vi "InsertAndPadVariantArrayBy1DIndex.vi"(9 "Array In":variant, 10 "Array Index (or -1)":i32, 11 "Value":variant) -> (3 "Reshaped VArray":variant)   [LabVIEW 2017]
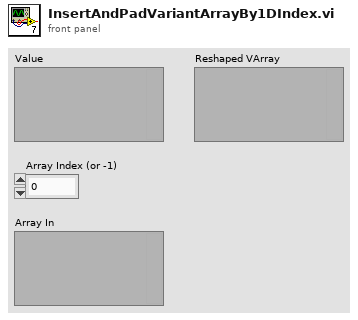
[diagram p1: front panel]
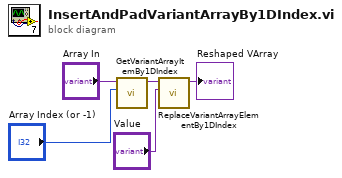
[diagram p0: block diagram]
diagram:
  n1 = call "GetVariantArrayItemBy1DIndex.vi"("Index"="Array Index (or -1)", "Array in"="Array In") -> ("Array out"=w2:variant)  [unwired: 8 in, 1 out]
  n2 = call "ReplaceVariantArrayElementBy1DIndex.vi"("Value"="Value", "Array in"=w2) -> ("Array out"=→"Reshaped VArray":variant)  [unwired: 9 in]
